vi "Pressure_Tapped_Cube.vi"(3 "Mode":T5, 5 "Traverse line In":T2 {"Row Duration (mins)" format="%#.1f"; "Row No" min=0; "Trace Gas Concentration (%)" min=0.0 format="%#.2f"; "Emission Rate (l/min)" format="%#.2f"; "Tunnel Speed" format="%#.2f"; "Start X" format="%#.2f"; "Start Y" format="%#.2f"; "Start Z" format="%#.2f"; "End X" format="%#.2f"; "End Y" format="%#.2f"; "End Z" format="%#.2f"; "Averaging time (min)" min=0.0 format="%#.1f"}) -> (0 "Error Message":string, 1 "Status":T1, 2 "Traverse line Out":T2 {"Row Duration (mins)" format="%#.1f"; "Row No" min=0; "Trace Gas Concentration (%)" min=0.0 format="%#.2f"; "Emission Rate (l/min)" format="%#.2f"; "Tunnel Speed" format="%#.2f"; "Start X" format="%#.2f"; "Start Y" format="%#.2f"; "Start Z" format="%#.2f"; "End X" format="%#.2f"; "End Y" format="%#.2f"; "End Z" format="%#.2f"; "Averaging time (min)" min=0.0 format="%#.1f"})   [LabVIEW 2010]
uses:
  Gen Trav/Traverse_cluster.ctl
  Gen Trav/Spacing.ctl
  Controls/Multi_run_mode.ctl
  Controls/User_Specific_mode.ctl
  Gen Trav/Multi_Run_Status.ctl
  Controls/Save_Data.ctl
  Controls/Setup.ctl
  Globals/Trav_pos_global.vi
  Globals/Meas_global.vi
  <vilib>/Analysis/NI_AALBase.lvlib
panel:
  out "XY Graph":cluster{dbl[], dbl[]}(graph)
  out "Measurement No":i32
  in  "stop":bool
  # "X           Y            Z"
  # "Start"
  # "End"
  # "X           Y            Z"
  # "Start"
  # "End"
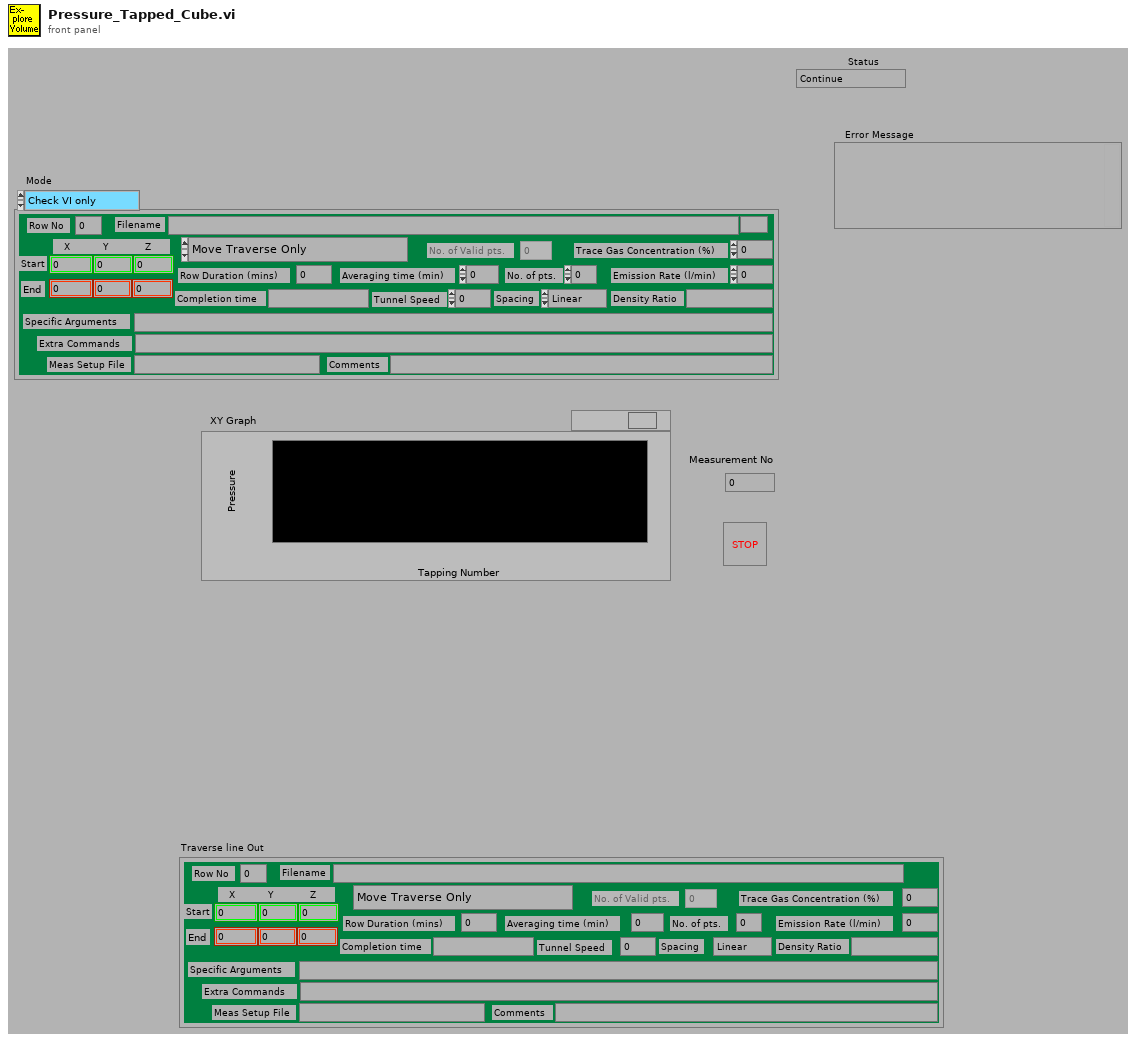
[diagram p1: front panel]
types:
  T1 = typedef "Multi_Run_Status.ctl" = enum16{"Continue", "Jump to Next Point", "Jump to Next Row", "Jump To Fall Back", "Terminate Run"}
  T2 = typedef "Traverse_cluster.ctl" = cluster{"Start X":dbl, "Start Y":dbl, "Start Z":dbl, "End X":dbl, "End Y":dbl, "End Z":dbl, "No. of pts.":i32, "Spacing":T3, "Filename":path, "Tunnel Speed":dbl, "Averaging time (min)":dbl, "Extra Commands":string, "Specific Arguments":string, "Emission Rate (l/min)":dbl, "Trace Gas Concentration (%)":dbl, "Density Ratio":string, "Comments":string, "Row No":i32, "Row Type Selector":T4, "Completion time":string, "Row Duration (mins)":dbl, "No. of Valid pts.":i32, "Meas Setup File":string}
  T3 = typedef "Spacing.ctl" = enum16{"Linear", "Log", "Gauss", "Specified", "N/A"}
  T4 = typedef "Multi_run_mode.ctl" = enum16{"Move Traverse Only", "Set Tunnel Speed Only", "Set Source Only", "Set Measurement Conditions", "Single Measurement", "Vertical Profile", "Lateral Profile", "Longitudinal Profile", "Explore Volume", "Multi-Axis Profile", "Auto Calibrate", "Meas Fast FID Bkgnd", "Check Beam Power", "Scanning Valve Measurement", "Run VI Named:", "Set ADAM Ch", "Wait (minutes)", "Send Message", "Synchronize With:", "Fall Back to this Row", "Turn Off Row Repeating", "Blank Row"}
  T5 = typedef "User_Specific_mode.ctl" = enum16{"Check VI only", "Run VI"}
  T6 = typedef "Save_Data.ctl" = enum16{"Save No Data", "Save Data"}
  T7 = typedef "Setup.ctl" = enum16{"Run Program", "Show Setup", "Save Current Setup", "Setup Front Panel"}
  T8 = cluster{"Name":string, "X":dbl, "Y":dbl, "Z":dbl}[]
  T9 = cluster{"Name":string, "X":dbl, "Y":dbl, "Z":dbl}
  T10 = typedef "Status_Cluster.ctl" = cluster{"Status":T1, "Error Type":string, "Error Description":string}
  T11 = typedef "Velocity_cluster.ctl" = cluster{"Name":string, "U":dbl, "u^2":dbl, "u^3/(u^2)^(1.5)":dbl, "u^4/(u^2)^2 -3":dbl, "% u'/U":dbl, "Mean % Err":dbl, "u^4":dbl}
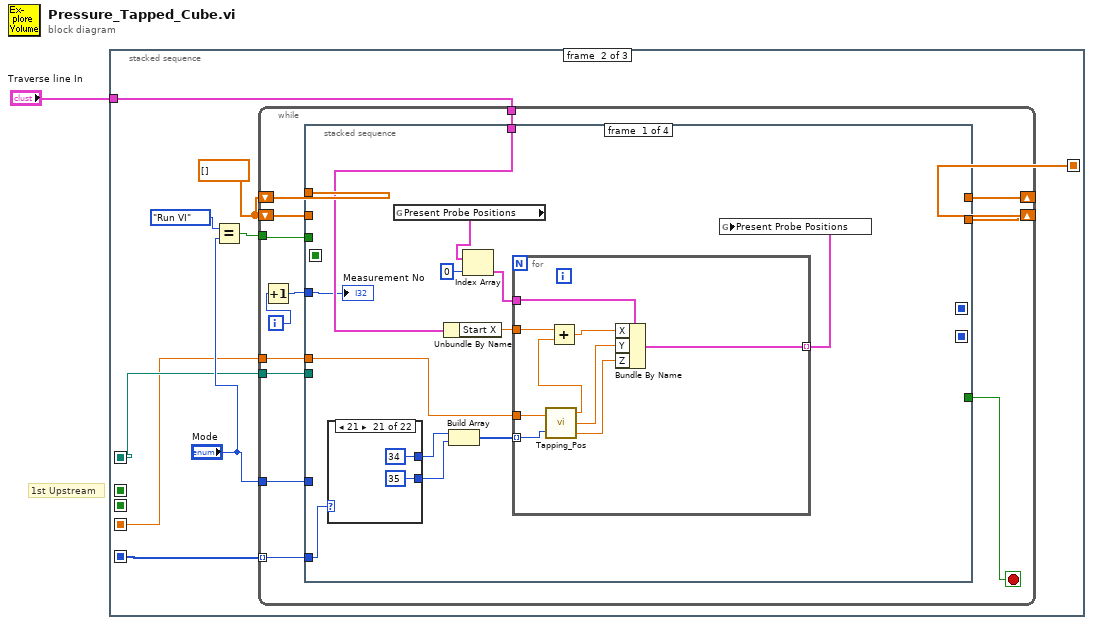
[diagram p0: block diagram]
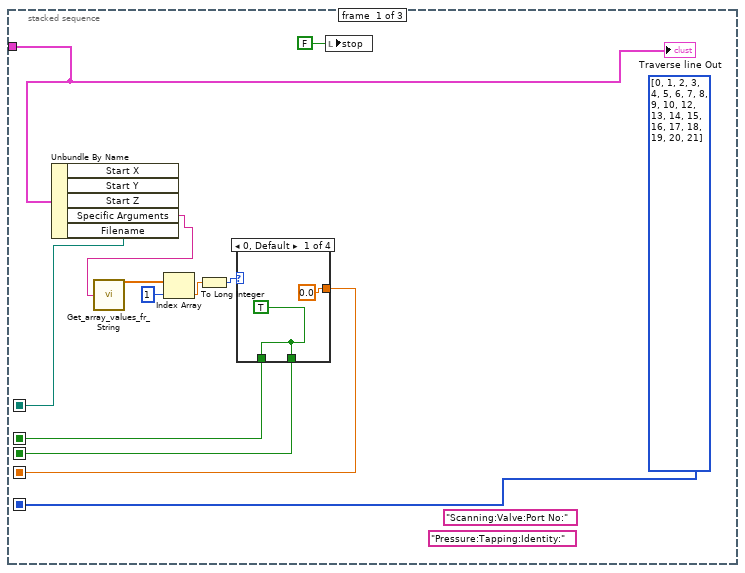
[diagram p2: hidden frame]
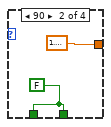
[diagram p3: hidden frame]
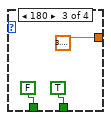
[diagram p4: hidden frame]
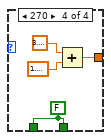
[diagram p5: hidden frame]
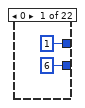
[diagram p6: hidden frame]
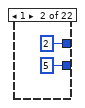
[diagram p7: hidden frame]
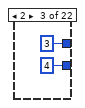
[diagram p8: hidden frame]
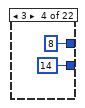
[diagram p9: hidden frame]
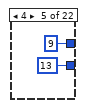
[diagram p10: hidden frame]
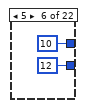
[diagram p11: hidden frame]
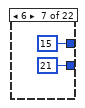
[diagram p12: hidden frame]
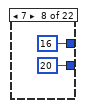
[diagram p13: hidden frame]
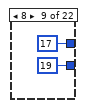
[diagram p14: hidden frame]
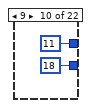
[diagram p15: hidden frame]
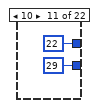
[diagram p16: hidden frame]
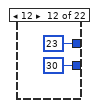
[diagram p17: hidden frame]
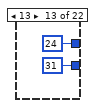
[diagram p18: hidden frame]
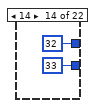
[diagram p19: hidden frame]
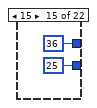
[diagram p20: hidden frame]
diagram:
  # "1st Upstream"
  n1 = stacked-sequence {
    seq-local: [w2 _ _] -> [_ w30 _]
    seq-local: [_ w29 _] -> [_ _ w221]
    seq-local: [w6 _ _] -> [_ _ w216]
    seq-local: [w4 _ _] -> [_ w26 _]
    seq-local: [w5 _ _] -> [_ _ w206]
    seq-local: [i32[] [0, 1, 2, 3, 4, 5, 6, 7, 8, 9, 10, 12, 13, 14, 15, 16, 17, 18, 19, 20, 21] _ _] -> [_ w25 _]
    tunnel: "Traverse line In" -> [w13 w27 _]
    frame #0 {
      (unwired) "Pressure:Tapping:Identity:"
      (unwired) "Scanning:Valve:Port No:"
      n2 = Unbundle By Name(w13) -> ("Specific Arguments"=w12:string, "Filename"=w2:path)  [unwired: 3 out]
      n3 = call "Get_array_values_fr_String.vi"("String Value"=w12) -> ("Numeric Array"=w10:dbl[])  [unwired: 1 out]
      n4 = Index Array(array=w10, index=1) -> (element=w8:dbl)
      n5 = To Long Integer(number=w8) -> (32bit integer=w7:i32)
      n6 = case shown="0, Default" w7 {
        tunnel: [0.0 1.5707963267948966 3.141592653589793 w22] -> w4
        tunnel: [w14 w16 FALSE w21] -> w6
        tunnel: [w14 w16 TRUE w21] -> w5
        frame 0, Default {
          w14 = TRUE
        }
        frame 90 {
          w16 = FALSE
        }
        frame 180 {
        }
        frame 270 {
          w21 = FALSE
          n7 = Add(x=3.141592653589793, y=1.5707963267948966) -> (x+y=w22:dbl)
        }
      }
      n8 = local write "stop"(FALSE ("stop")) -> ()
      "Traverse line Out" <- w13
    }
    frame #1 {
      w28 = dbl[] []
      n9 = Equal?(x=User_Specific_mode."Run VI" ("Mode"), y="Mode") -> (x = y?=w31:bool)
      n10 = while {
        tunnel: "Mode" -> [w41]
        tunnel: w31 -> [w37]
        tunnel: w30 -> [w46]
        shift-right: [w44] -> w29
        shift-left: w28 -> [w45]
        shift-right: [w42] -> _
        shift-left: w28 -> [w43]
        tunnel: w27 -> [w40]
        tunnel: w26 -> [w39]
        tunnel: w25 -> [w34] mode=indexing
        i -> [w36]
        stop <- w38 stop-if-true
        n11 = Increment(x=w36) -> (x+1=w35:i32)
        n12 = stacked-sequence {
          seq-local: [_ w114 _ _] -> [_ _ w142 _]
          seq-local: [_ w113 _ _] -> [_ _ w143 _]
          seq-local: [_ _ w144 _] -> [_ _ _ w198]
          tunnel: w46 -> [_ _ w150 _]
          tunnel: w45 -> [_ _ w149 _]
          tunnel: [_ _ w148 _] -> w44
          tunnel: w43 -> [_ _ w147 _]
          tunnel: [_ _ w146 _] -> w42
          tunnel: w41 -> [_ w117 _ _]
          tunnel: w40 -> [w58 w125 w145 _]
          tunnel: w35 -> [w52 _ _ w201]
          tunnel: w39 -> [w57 _ _ _]
          tunnel: [_ _ _ w199] -> w38
          tunnel: w37 -> [_ _ w141 _]
          tunnel: w34 -> [w47 w112 w139 _]
          frame #0 {
            n13 = case shown="21" w47 {
              tunnel: [1 2 3 8 9 10 15 16 17 11 22 23 24 32 36 37 39 41 26 28 34 -1] -> w56
              tunnel: [6 5 4 14 13 12 21 20 19 18 29 30 31 33 25 38 40 42 27 7 35 -1] -> w55
              frame 0 {
              }
              frame 1 {
              }
              frame 2 {
              }
              frame 3 {
              }
              frame 4 {
              }
              frame 5 {
              }
              frame 6 {
              }
              frame 7 {
              }
              frame 8 {
              }
              frame 9 {
              }
              frame 10 {
              }
              frame 12 {
              }
              frame 13 {
              }
              frame 14 {
              }
              frame 15 {
              }
              frame 16 {
              }
              frame 17 {
              }
              frame 18 {
              }
              frame 19 {
              }
              frame 20 {
              }
              frame 21 {
              }
              frame 22, Default {
              }
            }
            n14 = global read "Trav_pos_global.vi" "Present Probe Positions"() -> (w51:T8)
            n15 = Unbundle By Name(w58) -> ("Start X"=w53:dbl)
            n16 = Build Array(w56, w55) -> (w54:i32[])
            n17 = Index Array(array=w51, index=0) -> (element=w49:T9)
            n18 = for {
              tunnel: w57 -> [w111]
              tunnel: w54 -> [w110] mode=indexing
              tunnel: w53 -> [w109]
              tunnel: w49 -> [w105]
              tunnel: [w104] -> w48 mode=indexing
              n19 = call "Tapping_Pos.vi"("Orientation"=w111, "Tapping Number"=w110) -> ("X"=w108:dbl, "Y"=w103:dbl, "Z"=w106:dbl)
              n20 = Add(x=w109, y=w108) -> (x+y=w107:dbl)
              n21 = Bundle By Name(cluster=w105, "X"=w107, "Y"=w103, "Z"=w106) -> (w104:T9)
            }
            n22 = global write "Trav_pos_global.vi" "Present Probe Positions"(w48) -> ()
            "Measurement No" <- w52
          }
          frame #1 {
            n23 = case shown="\"Check VI only\", Default" w117 {
              tunnel: w112 -> [_ w129]
              tunnel: ["" w128] -> w118
              frame "Check VI only", Default {
              }
              frame "Run VI" {
                n24 = call "ScaniValve_client.vi"("Port Number"=w129) -> ("Error String"=w128:string)  [unwired: 2 out]
              }
            }
            n25 = Empty String/Path?(string/path=w118) -> (empty?=w121:bool)
            n26 = Not(x=w121) -> (.not. x?=w120:bool)
            n27 = Bundle By Name(cluster=w125, "Row Type Selector"=Multi_run_mode."Set Measurement Conditions", "Extra Commands"="!Skip Traverse Position Demand") -> (w122:T2)
            n28 = call "Set_Measurement_Conditions.vi"("Simulate/Run"=w117, "Currently on Point"=1, "Traverse line"=w122) -> ("Status Cluster"=w119:T10)  [unwired: 2 out]
            n29 = case shown="True" w120 {
              tunnel: w119 -> [w130 w138]
              tunnel: [w130 w135] -> w115
              tunnel: w118 -> [_ w132]
              tunnel: w112 -> [_ w131]
              frame False {
              }
              frame True {
                n30 = Format Into String(format string=" For Port No %d." ("Format String"), initial string=w132, w131) -> (resulting string=w133:string)  [unwired: 1 in, 1 out]
                n31 = Bundle By Name(cluster=w138, "Status"=Multi_Run_Status."Jump to Next Point", "Error Type"="Scanning Valve Error" ("t"), "Error Description"=w133) -> (w135:T10)
              }
            }
            n32 = Unbundle By Name(w115) -> ("Status"=w113:T1)
            n33 = Equal?(x=Multi_Run_Status."Continue" ("Status"), y=w113) -> (x = y?=w114:bool)
            n34 = call "Prog_Status_Handler.vi"("Status Cluster"=w115, "Simulate/Run"=w117) -> ()  [unwired: 2 out]
          }
          frame #2 {
            n35 = And(x=w141, y=w142) -> (x .and. y?=w140:bool)
            n36 = case shown="True" w140 {
              tunnel: [w151 w161] -> w144
              tunnel: w150 -> [_ w160]
              tunnel: w149 -> [w153 w159]
              tunnel: [w153 w158] -> w148
              tunnel: w147 -> [w152 w157]
              tunnel: [w152 w156] -> w146
              tunnel: w145 -> [_ w155]
              tunnel: w139 -> [_ w154]
              tunnel: w143 -> [w151 _]
              frame False {
                (unwired) FALSE ("stop")
              }
              frame True {
                n37 = stacked-sequence {
                  seq-local: [_ w173 _] -> [_ _ w189]
                  tunnel: [w164 _ _] -> w161
                  tunnel: w160 -> [w163 _ _]
                  tunnel: w159 -> [_ w174 _]
                  tunnel: [_ w173 _] -> w158
                  tunnel: w157 -> [_ _ w194]
                  tunnel: [_ _ w192] -> w156
                  tunnel: w155 -> [w162 _ _]
                  tunnel: w154 -> [_ _ w187]
                  frame #0 {
                    w167 = FALSE  # Acquisition Interlock
                    w168 = TRUE  # Open Front Panel
                    w170 = FALSE  # Remote control
                    n38 = Unbundle By Name(w162) -> ("Averaging time (min)"=w169:dbl)
                    n39 = call "Code_to_run.vi"("Open Front Panel"=w168, "Acquisition Interlock"=w167, "setup"=Setup."Run Program", "Remote control"=w170, "File"=Save_Data."Save Data", "Results Filename"=w163, "Averaging time (min)"=w169) -> ("Status"=w164:T1)  [unwired: 4 in, 4 out]
                  }
                  frame #1 {
                    n40 = global read "Meas_global.vi" "Velocity Cluster Array"() -> (w172:T11[])
                    n41 = Array Size(array=w172) -> (size(s)=w171:i32)
                    n42 = while {
                      tunnel: w172 -> [w186] mode=indexing
                      tunnel: [w184] -> _ mode=indexing
                      tunnel: [w185] -> w175
                      tunnel: w171 -> [w181]
                      i -> [w182]
                      stop <- w176 continue-if-true
                      n43 = Decrement(x=w181) -> (x-1=w180:i32)
                      n44 = Unbundle By Name(w186) -> ("Name"=w184:string, "U"=w185:dbl)
                      n45 = Match Pattern(string=w184, regular expression="Mano") -> (offset past match=w179:i32)  [unwired: 4 out]
                      n46 = Less?(x=w182, y=w180) -> (x < y?=w177:bool)
                      n47 = Less Than 0?(x=w179) -> (x < 0?=w178:bool)
                      n48 = And(x=w178, y=w177) -> (x .and. y?=w176:bool)
                    }
                    n49 = Build Array (concatenate)(w174, w175) -> (w173:dbl[])
                  }
                  frame #2 {
                    n50 = Build Array (concatenate)(w194, w187) -> (w192:dbl[])
                    n51 = call "Sort_Array_Indicies.vi"("unsorted array"=w192) -> ("sorted array"=w191:dbl[], "Sort Index"=w190:i32[])
                    n52 = for {
                      tunnel: w190 -> [w197] mode=indexing
                      tunnel: w189 -> [w196]
                      tunnel: [w195] -> w188 mode=indexing
                      n53 = Index Array(array=w196, index=w197) -> (element=w195:dbl)
                    }
                    n54 = Bundle("sorted array"=w191, w188) -> (→"XY Graph":cluster{"sorted array":dbl[], dbl[]})  [unwired: 1 out]
                  }
                }
              }
            }
          }
          frame #3 {
            n55 = Greater?(x=w198, y=Multi_Run_Status."Jump to Next Point" ("Status")) -> (0:w204:bool)
            n56 = Greater Or Equal?(x=w201, y=21.0) -> (x >= y?=w203:bool)
            n57 = Compound Arithmetic op=OR("stop", w204, w203) -> (w199:bool)
            "Status" <- w198
          }
        }
      }
    }
    frame #2 {
      n58 = Split 1D Array(array=w221, index=21) -> (first subarray=w219:dbl[], second subarray=w215:dbl[])
      n59 = Array Size(array=w215) -> (size(s)=w214:i32)
      n60 = call <vilib>:"Mean.vi"("X"=w219) -> ("mean"=w218:dbl)  [unwired: 1 out]
      n61 = call <vilib>:"Mean.vi"("X"=w215) -> ("mean"=w217:dbl)  [unwired: 1 out]
      n62 = Greater?(x=w214, y=19) -> (0:w207:bool)
      n63 = case shown="False" w216 {
        tunnel: w218 -> [w224 w227]
        tunnel: w217 -> [w223 w226]
        tunnel: [w222 w225] -> w212
        frame False {
          n64 = Greater?(x=w224, y=w223) -> (0:w222:bool)
        }
        frame True {
          n65 = Less?(x=w227, y=w226) -> (x < y?=w225:bool)
        }
      }
      n66 = Compound Arithmetic op=AND(w212, w207, w206) -> (w211:bool)
      n67 = Select(t="The Pressures on the upstream face are lower than the downstream face.\nMaybe you have incorrectly entered the orientation of the cube via the second specific argument.", s=w211, f="") -> (s? t:f=→"Error Message":string)
    }
  }
